vi "myRIO_BRig_RT_dataTrial_init.vi"() -> (3 "output_dataTrial":u16[][](array[numeric]))   [LabVIEW 2014]
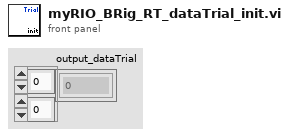
[diagram p1: front panel]
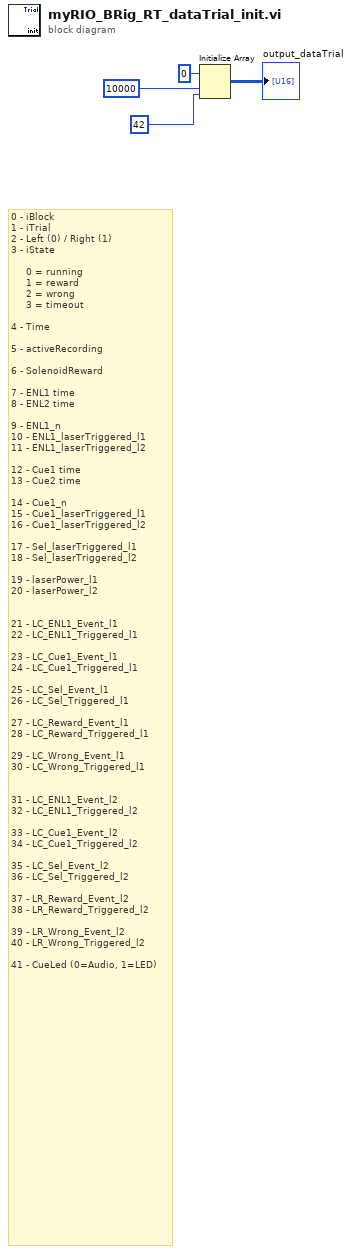
[diagram p0: block diagram]
diagram:
  # "0 - iBlock\n1 - iTrial\n2 - Left (0) / Right (1)\n3 - iState\n\n     0 = running\n     1 = reward\n     2 = wrong\n     3 = timeout\n\n4 - Time\n\n5 - activeRecording \n\n6 - SolenoidReward\n\n7 - ENL1 time\n8 - ENL2 time\n\n9 - ENL1_n\n10 - ENL1_laserTriggered_l1\n11 - ENL1_laserTriggered_l2\n\n12 - Cue1 time\n13 - Cue2 time\n\n14 - Cue1_n\n15 - Cue1_laserTriggered_l1\n16 - Cue1_laserTriggered_l2\n\n17 - Sel_laserTriggered_l1\n18 - Sel_laserTriggered_l2\n\n19 - laserPower_l1\n20 - laserPower_l2\n\n\n21 - LC_ENL1_Event_l1\n22 - LC_ENL1_Triggered_l1\n\n23 - LC_Cue1_Event_l1\n24 - LC_Cue1_Triggered_l1\n\n25 - LC_Sel_Event_l1\n26 - LC_Sel_Triggered_l1\n\n27 - LC_Reward_Event_l1\n28 - LC_Reward_Triggered_l1\n\n29 - LC_Wrong_Event_l1\n30 - LC_Wrong_Triggered_l1\n\n\n31 - LC_ENL1_Event_l2\n32 - LC_ENL1_Triggered_l2\n\n33 - LC_Cue1_Event_l2\n34 - LC_Cue1_Triggered_l2\n\n35 - LC_Sel_Event_l2\n36 - LC_Sel_Triggered_l2\n\n37 - LR_Reward_Event_l2\n38 - LR_Reward_Triggered_l2\n\n39 - LR_Wrong_Event_l2\n40 - LR_Wrong_Triggered_l2\n\n41 - CueLed (0=Audio, 1=LED)"
  n1 = Initialize Array(u16 0 ("element"), 10000 ("dimension size"), 42 ("dimension size")) -> (→"output_dataTrial":u16[][])
